vi "Throw Veristand Mapping Conflict Errors.vi"(7 "Type":T3, 8 "error in (no error)":errorcluster, 10 "Conflicts In":T1(array[cluster]), 11 "Item Ref in":T2 format="%.0x") -> (0 "error out":errorcluster, 2 "Conflicts?":bool, 3 "Node Ref out":T2 format="%.0x")   [LabVIEW 2015, in "Modbus Master System Explorer.lvlib"]
uses:
  Modbus Master System Explorer.lvlib
  Modbus Type.ctl
  <vilib>/NI Veristand/Custom Device API/Custom Device Item Ref.ctl
  <vilib>/NI VeriStand/Custom Device API/Custom Device API.lvlib
  Shared/Modbus Master Shared.lvlib
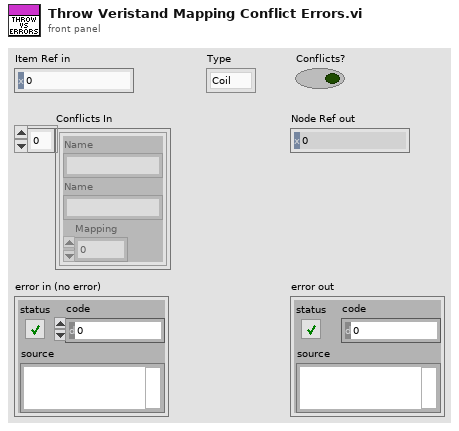
[diagram p1: front panel]
types:
  T1 = cluster{"Name":string, "Name":string, "Mapping":u16}[]
  T2 = typedef "Custom Device API.lvlib/Custom Device Item Ref.ctl" = u64
  T3 = typedef "Modbus Master Shared.lvlib/Modbus Type.ctl" = enum16{"Coil", "Discrete Input", "Holding Register", "Input Register"}
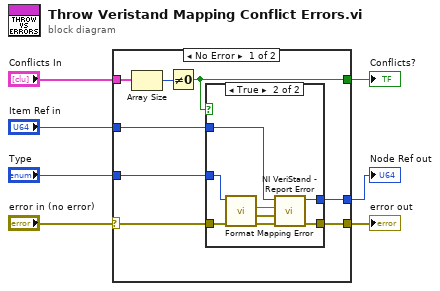
[diagram p0: block diagram]
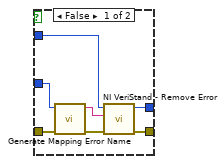
[diagram p2: hidden frame]
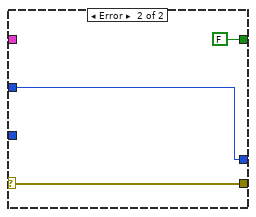
[diagram p3: hidden frame]
diagram:
  n1 = case shown="No Error" "error in (no error)" {
    selector: "error in (no error)" -> [w14 w33]
    tunnel: "Type" -> [w15 _]
    tunnel: [w13 w33] -> w5
    tunnel: [w12 w32] -> w4
    tunnel: "Item Ref in" -> [w11 w32]
    tunnel: [w10 FALSE] -> w2
    tunnel: "Conflicts In" -> [w9 _]
    frame No Error {
      n2 = Array Size(array=w9) -> (size(s)=w8:i32)
      n3 = Not Equal To 0?(x=w8) -> (x != 0?=w10:bool)
      n4 = case shown="True" w10 {
        tunnel: [w20 w30] -> w12
        tunnel: [w21 w29] -> w13
        tunnel: w11 -> [w22 w28]
        tunnel: w14 -> [w17 w27]
        tunnel: w15 -> [w18 w23]
        frame False {
          n5 = call "Generate Mapping Error Name.vi"("error in"=w17, "Type"=w18) -> ("error out"=w16:errorcluster, "String"=w19:string)  [unwired: 8 in]
          n6 = call <vilib>:"NI VeriStand - Remove Error.vi"("error in (no error)"=w16, "Error ID"=w19, "Node Ref in"=w22) -> ("error out"=w21:errorcluster, "Node Ref out"=w20:T2)  [unwired: 7 in]
        }
        frame True {
          n7 = call "Format Mapping Error.vi"("error in (no error)"=w27, "Type"=w23) -> ("error out"=w26:errorcluster, "mapping error out"=w25:errorcluster, "mapping error name"=w24:string)  [unwired: 7 in]
          n8 = call <vilib>:"NI VeriStand - Report Error.vi"("error in (no error)"=w26, "New Error"=w25, "Error ID"=w24, "Node Ref in"=w28) -> ("error out"=w29:errorcluster, "Node Ref out"=w30:T2)  [unwired: 6 in]
        }
      }
    }
    frame Error {
    }
  }
  "error out" <- w5
  "Node Ref out" <- w4
  "Conflicts?" <- w2
